vi "Find_Screen_Center.vi"() -> ()   [LabVIEW 2017]
uses:
  <vilib>/Utility/miscctls.llb/LVRectTypeDef.ctl
panel:
  in  "stop":bool
  out "Front Panel Window:Window Bounds":T1
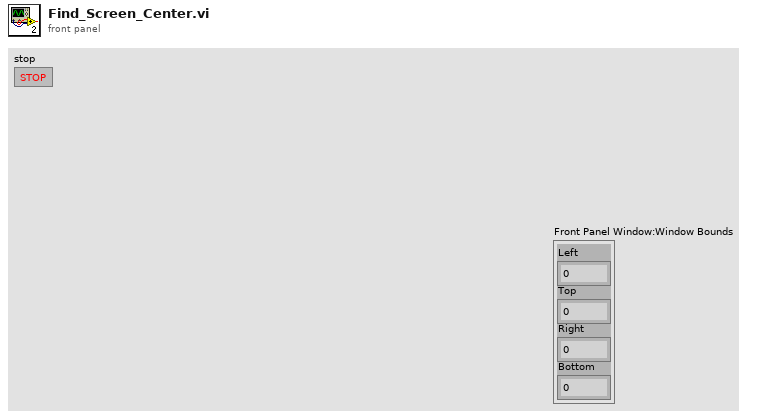
[diagram p1: front panel]
types:
  T1 = typedef "LVRectTypeDef.ctl" = cluster{"Left":i16, "Top":i16, "Right":i16, "Bottom":i16}
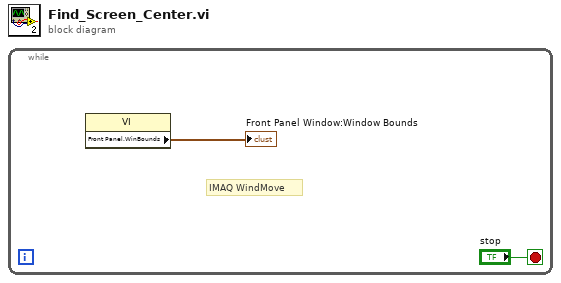
[diagram p0: block diagram]
diagram:
  n1 = while {
    stop <- "stop" stop-if-true
    # "IMAQ WindMove"
    n2 = property class="VI"() -> ("Front Panel.WinBounds"=→"Front Panel Window:Window Bounds":T1)  [unwired: 2 in, 2 out]
  }
